vi "Set_Joint_Configuration_Payload_EMG_Control.vi"(9 "EMG control":T1(ring), 10 "Current position":u16, 11 "Identifier selection in":u8) -> (3 "Set joint position command":T2 {"payload" format="%x"; "timestamp" format="%<%I:%M:%S%8u %p\n%x>T"; "identifier" format="%x"})   [LabVIEW 2015]
uses:
  <vilib>/Stratom, Inc/X-CAN for myRIO (API)/X-CAN Class/Type Definitions/CANFrame.ctl
  <vilib>/Stratom, Inc/X-CAN for myRIO (API)/X-CAN Class/X-CAN.lvclass
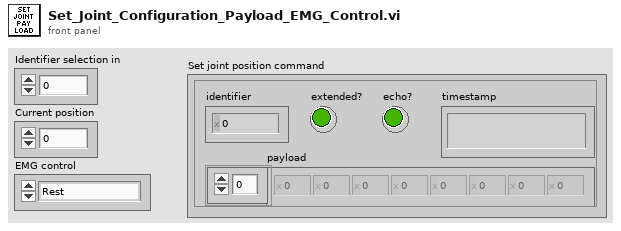
[diagram p1: front panel]
types:
  T1 = enum16{"Rest", "Biceps contracted", "Triceps contracted"}
  T2 = typedef "X-CAN.lvclass/CANFrame.ctl" = cluster{"identifier":u32, "extended?":bool, "echo?":bool, "payload":u8[], "timestamp":timestamp}
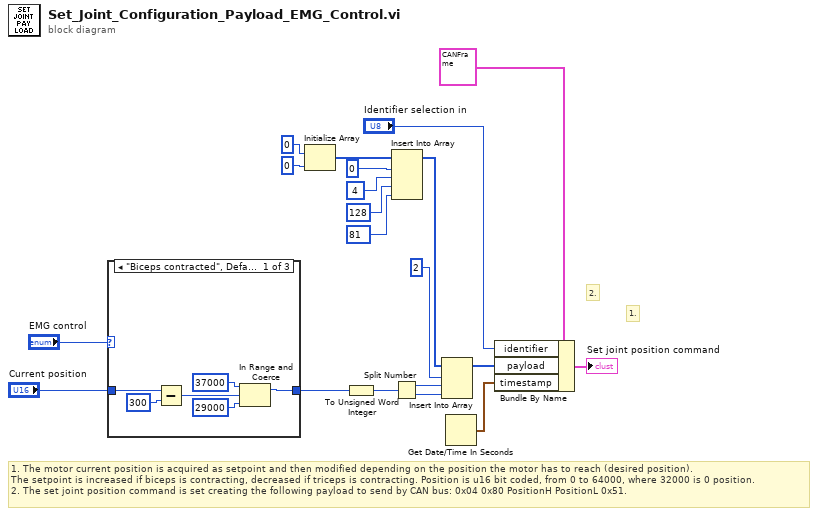
[diagram p0: block diagram]
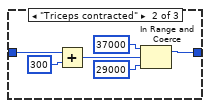
[diagram p2: hidden frame]
diagram:
  # "1."
  # "2."
  # "1. The motor current position is acquired as setpoint and then modified depending on the position the motor has to reach (desired position).\nThe setpoint is increased if biceps is contracting, decreased if triceps is contracting. Position is u16 bit coded, from 0 to 64000, where 32000 is 0 position.\n2. The set joint position command is set creating the following payload to send by CAN bus: 0x04 0x80 PositionH PositionL 0x51."
  n1 = case shown="\"Biceps contracted\", Default" "EMG control" {
    tunnel: "Current position" -> [w26 w32 w33]
    tunnel: [w23 w27 w33] -> w3
    frame "Biceps contracted", Default {
      n2 = Subtract(x=w26, y=u16 300 ("x")) -> (x-y=w24:u16)
      n3 = In Range and Coerce(upper limit=u16 37000, x=w24, lower limit=u16 29000) -> (coerced(x)=w23:u16)  [unwired: 1 out]
    }
    frame "Triceps contracted" {
      n4 = Add(x=w32, y=u16 300) -> (x+y=w28:u16)
      n5 = In Range and Coerce(upper limit=u16 37000, x=w28, lower limit=u16 29000) -> (coerced(x)=w27:u16)  [unwired: 1 out]
    }
    frame "Rest" {
    }
  }
  n6 = Initialize Array(u16 0 ("element"), 0 ("dimension size")) -> (w11:u16[])
  n7 = To Unsigned Word Integer(number=w3) -> (unsigned 16bit integer=w20:u16)
  n8 = Insert Into Array(array=w11, index=0, new element #1=u8 4 ("new element/subarray"), new element #2=u8 128 ("new element/subarray"), new element #3=u8 81 ("new element/subarray")) -> (w7:u16[])
  n9 = Split Number(x=w20) -> (hi(x)=w17:u8, lo(x)=w16:u8)
  n10 = Insert Into Array(array=w7, index=2, new element #1=w17, new element #2=w16) -> (w14:u16[])
  n11 = Get Date/Time In Seconds() -> (seconds since 1Jan1904=w6:timestamp)
  n12 = Bundle By Name(cluster=T2 {"identifier"=0, "extended?"=FALSE, "echo?"=FALSE, "payload"=[], "timestamp"=timestamp(0 s since 1904-01-01)} ("CAN Frame"), "identifier"="Identifier selection in", "payload"=w14, "timestamp"=w6) -> (→"Set joint position command":T2)
